vi "Modify ZPL File Label.vi"(1 "HW version":string, 2 "SW version":string, 5 "error in":errorcluster, 6 "Variant":string) -> (19 "error out":errorcluster)   [LabVIEW 2023]
panel:
  out "resulting string":string
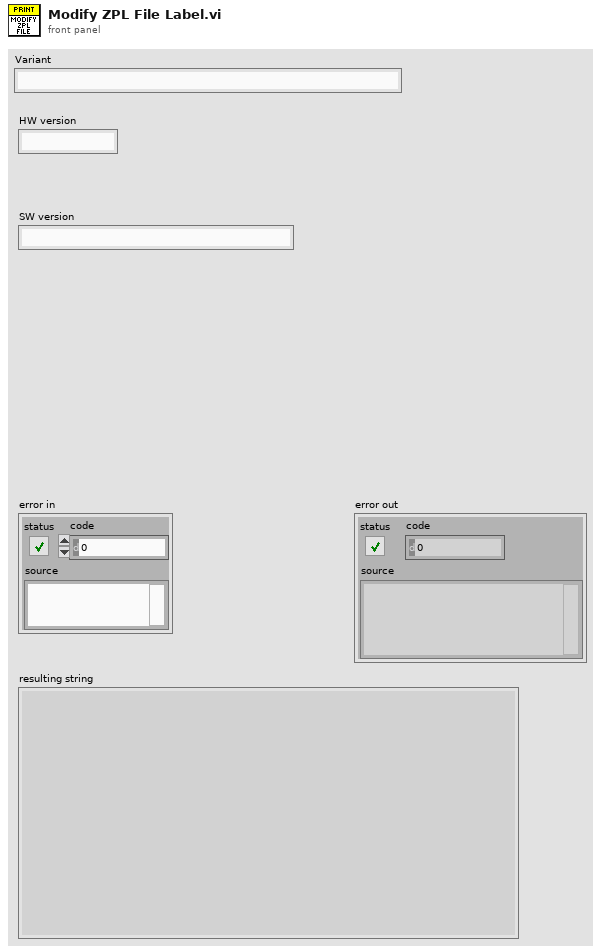
[diagram p1: front panel]
types:
  T1 = enum16{"open", "replace", "create", "open or create", "replace or create", "replace or create with confirmation"}
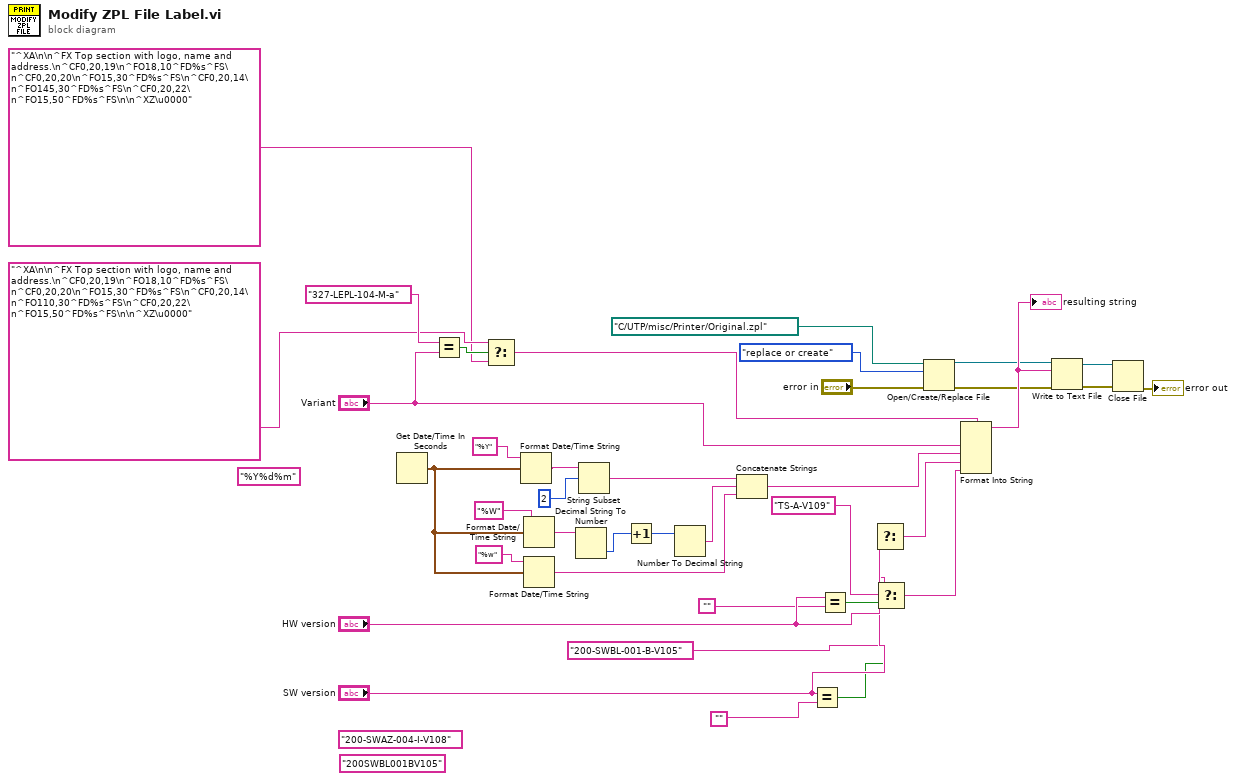
[diagram p0: block diagram]
diagram:
  (unwired) "%Y%d%m" ("time format string (%c)")
  (unwired) "200-SWAZ-004-I-V108"
  (unwired) "200SWBL001BV105"
  n1 = Get Date/Time In Seconds() -> (seconds since 1Jan1904=w22:timestamp)
  n2 = Equal?(x="327-LEPL-104-M-a", y="Variant") -> (x = y?=w9:bool)
  n3 = Select(t="^XA\n\n^FX Top section with logo, name and address.\n^CF0,20,19\n^FO18,10^FD%s^FS\n^CF0,20,20\n^FO15,30^FD%s^FS\n^CF0,20,14\n^FO110,30^FD%s^FS\n^CF0,20,22\n^FO15,50^FD%s^FS\n\n^XZ\u0000" ("format string"), s=w9, f="^XA\n\n^FX Top section with logo, name and address.\n^CF0,20,19\n^FO18,10^FD%s^FS\n^CF0,20,20\n^FO15,30^FD%s^FS\n^CF0,20,14\n^FO145,30^FD%s^FS\n^CF0,20,22\n^FO15,50^FD%s^FS\n\n^XZ\u0000" ("format string")) -> (s? t:f=w1:string)
  n4 = Format Date/Time String(time format string (%c)="%Y", seconds (now)=w22) -> (date/time string=w37:string)  [unwired: 1 in]
  n5 = Format Date/Time String(time format string (%c)="%W", seconds (now)=w22) -> (date/time string=w21:string)  [unwired: 1 in]
  n6 = Format Date/Time String(time format string (%c)="%w", seconds (now)=w22) -> (date/time string=w13:string)  [unwired: 1 in]
  n7 = Decimal String To Number(string=w21) -> (number=w20:i32)  [unwired: 2 in, 1 out]
  n8 = String Subset(string=w37, offset (0)=2) -> (substring=w15:string)  [unwired: 1 in]
  n9 = Increment(x=w20) -> (x+1=w19:i32)
  n10 = Number To Decimal String(number=w19) -> (decimal integer string=w14:string)  [unwired: 1 in]
  n11 = Concatenate Strings(w15, w14, w13) -> (w12:string)
  n12 = Equal?(x="SW version", y="") -> (x = y?=w26:bool)
  n13 = Equal?(x="HW version", y="") -> (x = y?=w28:bool)
  n14 = Select(t="TS-A-V109", s=w28, f="HW version") -> (s? t:f=w17:string)
  n15 = Select(t="200-SWBL-001-B-V105", s=w26, f="SW version") -> (s? t:f=w16:string)
  n16 = Open/Create/Replace File(file path (use dialog)=path "C:/UTP/misc/Printer/Original.zpl", error in="error in", operation (0:open)=T1."replace or create") -> (refnum out=w5:refnum<file>, error out=w4:errorcluster)  [unwired: 3 in, 1 out]
  n17 = Format Into String(format string=w1, "Variant", w12, w17, w16) -> (resulting string=w18:string)  [unwired: 2 in, 1 out]
  "resulting string" <- w18
  n18 = Write to Text File(file (use dialog)=w5, text=w18, error in=w4) -> (refnum out=w6:refnum<file>, error out=w3:errorcluster)  [unwired: 1 in, 1 out]
  n19 = Close File(refnum=w6, error in=w3) -> (error out=→"error out":errorcluster)  [unwired: 1 out]
